vi "Subsys01_Main.vi"() -> ()   [LabVIEW 2019]
uses:
  Subsys01_Global.vi
panel:
  out "status":u32(colorbox)
  out "value":dbl
  out "spill_id_global":i64
  in  "stop":bool
  out "spill_id":i64
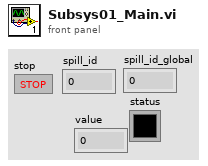
[diagram p1: front panel]
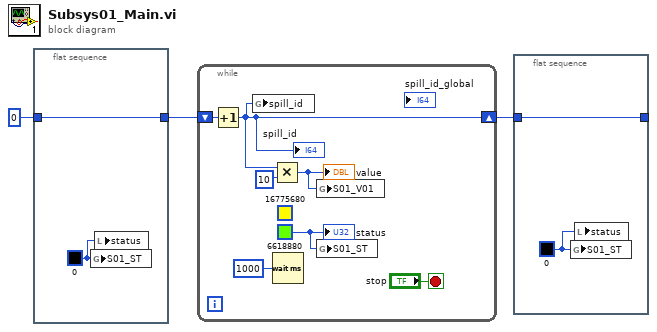
[diagram p0: block diagram]
diagram:
  n1 = flat-sequence {
    tunnel: 0 -> [w5]
    tunnel: [w5] -> w2
    frame #0 {
      w4 = u32 0 ("alarm_status")
      n2 = global write "Subsys01_Global.vi" "S01_ST"(w4) -> ()
      n3 = local write "status"(w4) -> ()
    }
  }
  n4 = while {
    shift-right: [w9] -> w1
    shift-left: w2 -> [w12]
    stop <- "stop" stop-if-true
    (unwired) u32 16775680 ("alarm_status")
    w6 = u32 6618880 ("alarm_status")
    n5 = Increment(x=w12) -> (x+1=w9:i32)
    "spill_id" <- w9
    n6 = global write "Subsys01_Global.vi" "spill_id"(w9) -> ()
    n7 = Multiply(x=w9, y=10) -> (x*y=w7:i32)
    "value" <- w7
    n8 = Wait (ms)(milliseconds to wait=u32 1000) -> ()  [unwired: 1 out]
    n9 = global write "Subsys01_Global.vi" "S01_V01"(w7) -> ()
    n10 = global write "Subsys01_Global.vi" "S01_ST"(w6) -> ()
    "status" <- w6
  }
  n11 = flat-sequence {
    tunnel: w1 -> [w14]
    tunnel: [w14] -> _
    frame #0 {
      w13 = u32 0 ("alarm_status")
      n12 = global write "Subsys01_Global.vi" "S01_ST"(w13) -> ()
      n13 = local write "status"(w13) -> ()
    }
  }
